vi "BRig_RT_panel_cue_v0,90.vi"(7 "input_setValues":bool, 11 "input_dataExp":u16[](array[numeric])) -> (3 "output_dataExp":u16[](array[numeric]))   [LabVIEW 2014]
panel:
  in  "CueLed_baseline":bool
  in  "CueSwitch_Count_PostR":u16
  in  "CueSwitch_Prob_PostR":u16
  in  "CueSwitch_PostR":u16(slide) max=3 step=1 scale=0.0..3.0
  in  "CueSwitch_Count_PreR":u16
  in  "CueSwitch_Count_First":u16
  in  "CueSwitch_Prob_PreR":u16
  in  "CueSwitch_PreR":u16(slide) max=3 step=1 scale=0.0..3.0
  in  "CueSwitch_Prob_First":u16
  in  "CueSwitch_First":u16(slide) max=3 step=1 scale=0.0..3.0
  in  "CueLed_Freq":u16=10
  in  "CueLed_Tpeak":u16=2
  in  "sp_RightSpout":u16(slide)=2 max=2 step=1 scale=0.0..2.0
  in  "sp_LeftSpout":u16(slide)=2 max=2 step=1 scale=0.0..2.0
  in  "Audio_Amp__R":u16=100 caption="Amp"
  in  "Audio_Freq__R":u16=5 caption="Freq [kHz]" max=14 step=1
  in  "Audio_Amp__L":u16=100 caption="Amp"
  in  "Audio_Freq__L":u16=5 caption="Freq [kHz]" max=14 step=1
  # "Cue State\n                                  Cue Type           LED Probability [%]      Count"
  # "Audio or LED"
  # "First"
  # "Pre Reward"
  # "Post Reward"
  # "Audio Parameters"
  # "Cue LED Parameters"
  # "Left                  Right"
  # "Frequency\n[Hz]"
  # "Frequency\n[kHz]"
  # "Timing [ms]\n                    Peak Width"
  # "Amp\n(0 - 32,000)"
  # "Speaker\nPattern\nDuring Cue"
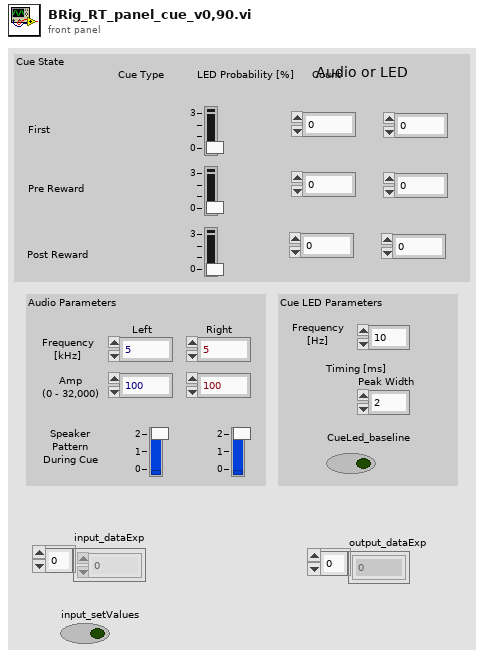
[diagram p1: front panel]
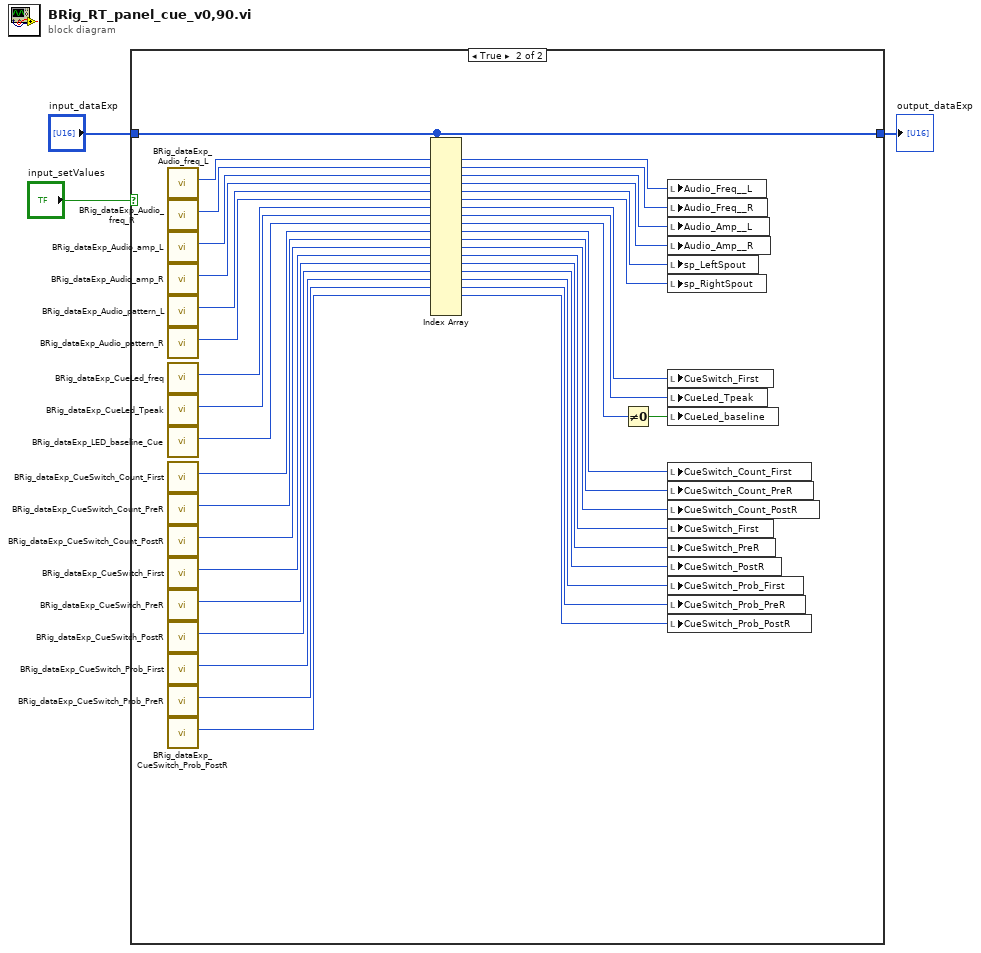
[diagram p0: block diagram]
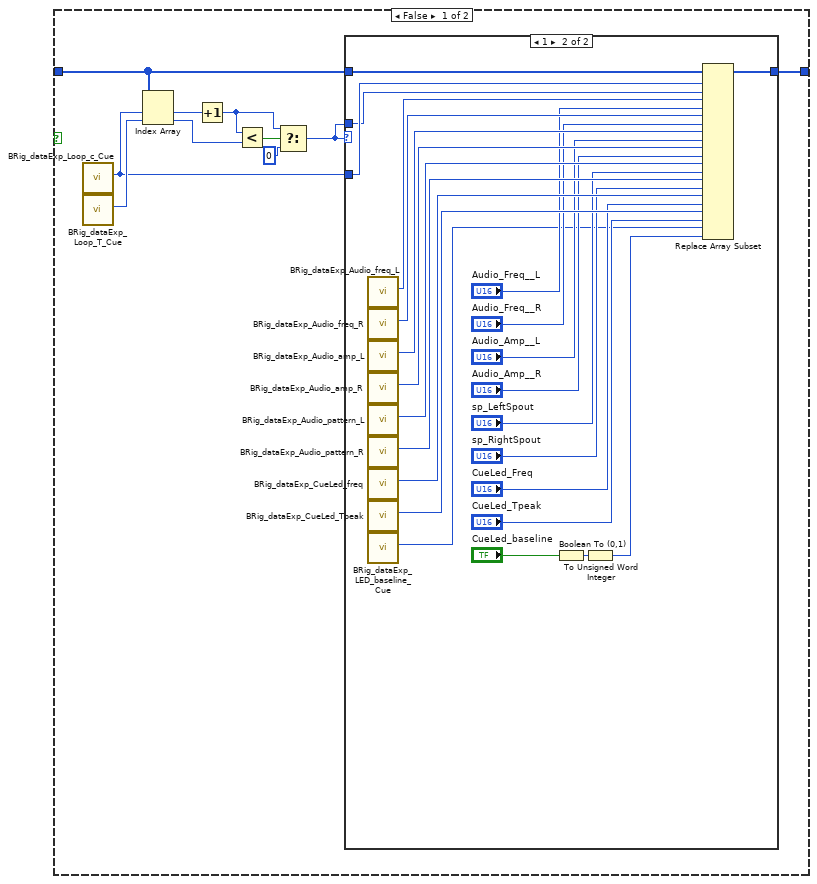
[diagram p2: hidden frame]
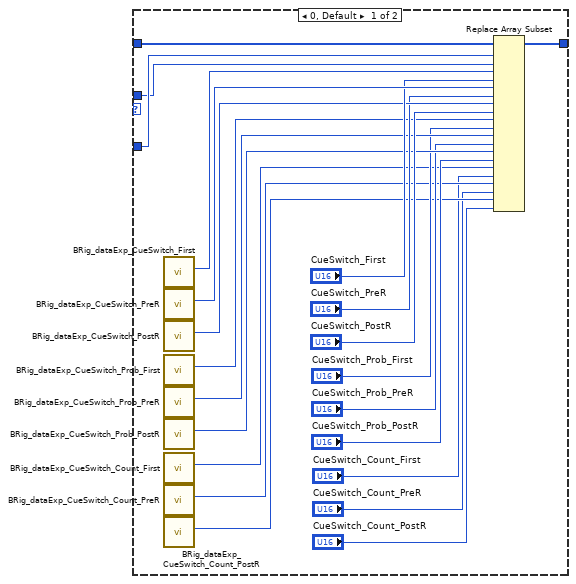
[diagram p3: hidden frame]
diagram:
  n1 = case shown="True" "input_setValues" {
    tunnel: "input_dataExp" -> [w7 w97]
    tunnel: [w6 w97] -> w2
    frame False {
      n2 = call "BRig_dataExp_Loop_c_Cue.vi"() -> ("output_Loop_c_Cue"=w5:i32)  [unwired: 11 in]
      n3 = call "BRig_dataExp_Loop_T_Cue.vi"() -> ("output_Loop_T_Cue"=w13:i32)  [unwired: 11 in]
      n4 = Index Array(array=w7, index #1=w5, index #2=w13) -> (element #1=w12:u16, element #2=w11:u16)
      n5 = Increment(x=w12) -> (x+1=w9:u16)
      n6 = Less?(x=w9, y=w11) -> (x < y?=w10:bool)
      n7 = Select(t=w9, s=w10, f=u16 0) -> (s? t:f=w4:u16)
      n8 = case shown="1" w4 {
        tunnel: w7 -> [w35 w59]
        tunnel: [w16 w58] -> w6
        tunnel: w5 -> [w15 w57]
        tunnel: w4 -> [w14 w56]
        frame 0, Default {
          n9 = call "BRig_dataExp_CueSwitch_First.vi"() -> ("output_CueSwitch_First"=w34:i32)  [unwired: 11 in]
          n10 = call "BRig_dataExp_CueSwitch_PreR.vi"() -> ("output_CueSwitch_PreR"=w33:i32)  [unwired: 11 in]
          n11 = call "BRig_dataExp_CueSwitch_PostR.vi"() -> ("output_CueSwitch_PostR"=w31:i32)  [unwired: 11 in]
          n12 = call "BRig_dataExp_CueSwitch_Prob_First.vi"() -> ("output_CueSwitch_Prob_First"=w28:i32)  [unwired: 11 in]
          n13 = call "BRig_dataExp_CueSwitch_Prob_PreR.vi"() -> ("output_CueSwitch_Prob_PreR"=w27:i32)  [unwired: 11 in]
          n14 = call "BRig_dataExp_CueSwitch_Prob_PostR.vi"() -> ("output_CueSwitch_Prob_PostR"=w26:i32)  [unwired: 11 in]
          n15 = call "BRig_dataExp_CueSwitch_Count_First.vi"() -> ("output_CueSwitch_Count_First"=w22:i32)  [unwired: 11 in]
          n16 = call "BRig_dataExp_CueSwitch_Count_PreR.vi"() -> ("output_CueSwitch_Count_PreR"=w21:i32)  [unwired: 11 in]
          n17 = call "BRig_dataExp_CueSwitch_Count_PostR.vi"() -> ("output_CueSwitch_Count_PostR"=w20:i32)  [unwired: 11 in]
          n18 = Replace Array Subset(array=w35, new element #1=w14, index #1=w15, new element #2="CueSwitch_First", index #2=w34, new element #3="CueSwitch_PreR", index #3=w33, new element #4="CueSwitch_PostR", index #4=w31, new element #5="CueSwitch_Prob_First", index #5=w28, new element #6="CueSwitch_Prob_PreR", index #6=w27, new element #7="CueSwitch_Prob_PostR", index #7=w26, new element #8="CueSwitch_Count_First", index #8=w22, new element #9="CueSwitch_Count_PreR", index #9=w21, new element #10="CueSwitch_Count_PostR", index #10=w20) -> (w16:u16[])
        }
        frame 1 {
          n19 = call "BRig_dataExp_Audio_freq_L.vi"() -> ("output_Audio_freq__L"=w55:i32)  [unwired: 11 in]
          n20 = call "BRig_dataExp_Audio_freq_R.vi"() -> ("output_Audio_freq__R"=w54:i32)  [unwired: 11 in]
          n21 = call "BRig_dataExp_Audio_amp_L.vi"() -> ("output_Audio_amp__L"=w53:i32)  [unwired: 11 in]
          n22 = call "BRig_dataExp_Audio_amp_R.vi"() -> ("output_Audio_amp__R"=w52:i32)  [unwired: 11 in]
          n23 = call "BRig_dataExp_Audio_pattern_L.vi"() -> ("output_Audio_sp__L"=w51:i32)  [unwired: 11 in]
          n24 = call "BRig_dataExp_Audio_pattern_R.vi"() -> ("output_Audio_sp__R"=w50:i32)  [unwired: 11 in]
          n25 = call "BRig_dataExp_CueLed_freq.vi"() -> ("output_CueLed_Freq"=w49:i32)  [unwired: 11 in]
          n26 = call "BRig_dataExp_CueLed_Tpeak.vi"() -> ("output_CueLed_Tpeak"=w48:i32)  [unwired: 11 in]
          n27 = call "BRig_dataExp_LED_baseline_Cue.vi"() -> ("output_LED_baseline_Cue"=w39:i32)  [unwired: 11 in]
          n28 = Boolean To (0,1)(Boolean="CueLed_baseline") -> (0, 1=w37:i16)
          n29 = To Unsigned Word Integer(number=w37) -> (unsigned 16bit integer=w36:u16)
          n30 = Replace Array Subset(array=w59, new element #1=w56, index #1=w57, new element #2="Audio_Freq__L", index #2=w55, new element #3="Audio_Freq__R", index #3=w54, new element #4="Audio_Amp__L", index #4=w53, new element #5="Audio_Amp__R", index #5=w52, new element #6="sp_LeftSpout", index #6=w51, new element #7="sp_RightSpout", index #7=w50, new element #8="CueLed_Freq", index #8=w49, new element #9="CueLed_Tpeak", index #9=w48, new element #10=w36, index #10=w39) -> (w58:u16[])
        }
      }
    }
    frame True {
      n31 = call "BRig_dataExp_Audio_freq_L.vi"() -> ("output_Audio_freq__L"=w96:i32)  [unwired: 11 in]
      n32 = call "BRig_dataExp_Audio_freq_R.vi"() -> ("output_Audio_freq__R"=w94:i32)  [unwired: 11 in]
      n33 = call "BRig_dataExp_Audio_amp_L.vi"() -> ("output_Audio_amp__L"=w92:i32)  [unwired: 11 in]
      n34 = call "BRig_dataExp_Audio_amp_R.vi"() -> ("output_Audio_amp__R"=w90:i32)  [unwired: 11 in]
      n35 = call "BRig_dataExp_Audio_pattern_L.vi"() -> ("output_Audio_sp__L"=w88:i32)  [unwired: 11 in]
      n36 = call "BRig_dataExp_Audio_pattern_R.vi"() -> ("output_Audio_sp__R"=w87:i32)  [unwired: 11 in]
      n37 = call "BRig_dataExp_CueLed_freq.vi"() -> ("output_CueLed_Freq"=w84:i32)  [unwired: 11 in]
      n38 = call "BRig_dataExp_CueLed_Tpeak.vi"() -> ("output_CueLed_Tpeak"=w82:i32)  [unwired: 11 in]
      n39 = call "BRig_dataExp_LED_baseline_Cue.vi"() -> ("output_LED_baseline_Cue"=w80:i32)  [unwired: 11 in]
      n40 = call "BRig_dataExp_CueSwitch_Count_First.vi"() -> ("output_CueSwitch_Count_First"=w77:i32)  [unwired: 11 in]
      n41 = call "BRig_dataExp_CueSwitch_Count_PreR.vi"() -> ("output_CueSwitch_Count_PreR"=w76:i32)  [unwired: 11 in]
      n42 = call "BRig_dataExp_CueSwitch_Count_PostR.vi"() -> ("output_CueSwitch_Count_PostR"=w75:i32)  [unwired: 11 in]
      n43 = call "BRig_dataExp_CueSwitch_First.vi"() -> ("output_CueSwitch_First"=w74:i32)  [unwired: 11 in]
      n44 = call "BRig_dataExp_CueSwitch_PreR.vi"() -> ("output_CueSwitch_PreR"=w73:i32)  [unwired: 11 in]
      n45 = call "BRig_dataExp_CueSwitch_PostR.vi"() -> ("output_CueSwitch_PostR"=w72:i32)  [unwired: 11 in]
      n46 = call "BRig_dataExp_CueSwitch_Prob_First.vi"() -> ("output_CueSwitch_Prob_First"=w71:i32)  [unwired: 11 in]
      n47 = call "BRig_dataExp_CueSwitch_Prob_PreR.vi"() -> ("output_CueSwitch_Prob_PreR"=w70:i32)  [unwired: 11 in]
      n48 = call "BRig_dataExp_CueSwitch_Prob_PostR.vi"() -> ("output_CueSwitch_Prob_PostR"=w69:i32)  [unwired: 11 in]
      n49 = Index Array(array=w97, index #1=w96, index #2=w94, index #3=w92, index #4=w90, index #5=w88, index #6=w87, index #7=w84, index #8=w82, index #9=w80, index #10=w77, index #11=w76, index #12=w75, index #13=w74, index #14=w73, index #15=w72, index #16=w71, index #17=w70, index #18=w69) -> (element #1=w95:u16, element #2=w93:u16, element #3=w91:u16, element #4=w89:u16, element #5=w86:u16, element #6=w85:u16, element #7=w83:u16, element #8=w81:u16, element #9=w78:u16, element #10=w68:u16, element #11=w67:u16, element #12=w66:u16, element #13=w65:u16, element #14=w64:u16, element #15=w63:u16, element #16=w62:u16, element #17=w61:u16, element #18=w60:u16)  [unwired: 2 in, 2 out]
      n50 = Not Equal To 0?(x=w78) -> (x != 0?=w79:bool)
      n51 = local write "Audio_Freq__L"(w95) -> ()
      n52 = local write "Audio_Freq__R"(w93) -> ()
      n53 = local write "Audio_Amp__L"(w91) -> ()
      n54 = local write "Audio_Amp__R"(w89) -> ()
      n55 = local write "sp_LeftSpout"(w86) -> ()
      n56 = local write "sp_RightSpout"(w85) -> ()
      n57 = local write "CueSwitch_First"(w83) -> ()
      n58 = local write "CueLed_Tpeak"(w81) -> ()
      n59 = local write "CueLed_baseline"(w79) -> ()
      n60 = local write "CueSwitch_Count_First"(w68) -> ()
      n61 = local write "CueSwitch_Count_PreR"(w67) -> ()
      n62 = local write "CueSwitch_Count_PostR"(w66) -> ()
      n63 = local write "CueSwitch_First"(w65) -> ()
      n64 = local write "CueSwitch_PreR"(w64) -> ()
      n65 = local write "CueSwitch_PostR"(w63) -> ()
      n66 = local write "CueSwitch_Prob_First"(w62) -> ()
      n67 = local write "CueSwitch_Prob_PreR"(w61) -> ()
      n68 = local write "CueSwitch_Prob_PostR"(w60) -> ()
    }
  }
  "output_dataExp" <- w2
